vi "Create Evaluation String.vi"(8 "error in (no error)":errorcluster, 10 "Evaluation String":string, 11 "FP Equal in":refnum<class "FP Equal.lvclass">) -> (0 "error out":errorcluster, 3 "FP Equal out":refnum<class "FP Equal.lvclass">)   [LabVIEW 2018, in "FP Equal.lvclass"]
uses:
  FP Equal.lvclass
  C:/Users/UKHornP/Documents/Work/Projects/Assert_API/Plugins/Utility/Test Classes/Test.lvclass
  FP Equal.lvclass/FP Equal.ctl
  Floating Point.lvclass
  Test.lvclass
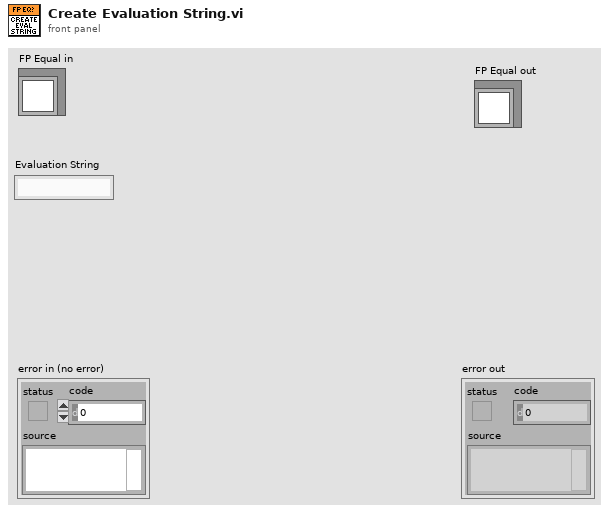
[diagram p1: front panel]
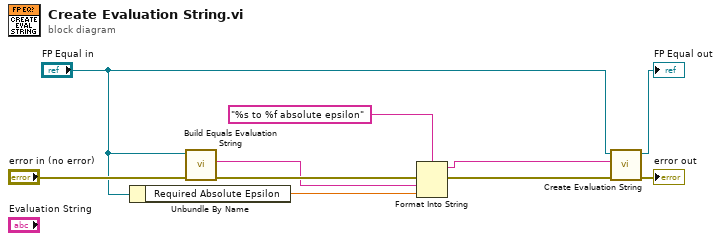
[diagram p0: block diagram]
diagram:
  n1 = Unbundle By Name("FP Equal in") -> ("Required Absolute Epsilon"=w2:dbl)
  n2 = call "Build Equals Evaluation String.vi"("error in (no error)"="error in (no error)", "Test in"="FP Equal in") -> ("error out"=w7:errorcluster, "Equals Evaluation String"=w3:string)  [unwired: 8 in]
  n3 = Format Into String(format string="%s to %f absolute epsilon", error in=w7, w3, w2) -> (resulting string=w4:string, error out=w5:errorcluster)  [unwired: 1 in]
  n4 = call-parent "Create Evaluation String.vi"("error in (no error)"=w5, "Evaluation String"=w4, "Floating Point in"="FP Equal in") -> ("error out"=→"error out":errorcluster, "Floating Point out"=→"FP Equal out":refnum<class "FP Equal.lvclass">)  [unwired: 7 in]
